vi "Poll PDOs.vi"(0 "interface object in":refnum<k20>, 1 "node-ID":u8=1, 11 "error in (no error)":errorcluster) -> (4 "PDO 1":u8[](array[numeric]), 6 "PDO 2":u8[](array[numeric]), 8 "PDO 3":u8[](array[numeric]), 10 "PDO 4":u8[](array[numeric]), 15 "error out":errorcluster)   [LabVIEW 2016]
uses:
  <vilib>/Platform/TimedLoop/XDataNode/timing_clust.ctl
  <vilib>/Platform/TimedLoop/XDataNode/nitl_modes.ctl
  <vilib>/Platform/TimedLoop/XDataNode/wakeup.ctl
  <vilib>/CANopenLib/CANOPEN.llb/CANopen SYNC Create.vi
  <vilib>/CANopenLib/CANOPEN.llb/CANopen SYNC Start.vi
  <vilib>/CANopenLib/CANOPEN.llb/CANopen TPDO Create.vi
  <vilib>/CANopenLib/CANOPEN.llb/CANopen TPDO Start.vi
  <vilib>/CANopenLib/CANOPEN.llb/CANopen SYNC Close.vi
  <vilib>/CANopenLib/CANOPEN.llb/CANopen TPDO Close.vi
  <vilib>/Platform/TimedLoop/XDataNode/XDataNode.xnode
  <vilib>/Platform/TimedLoop/XDataNode/XDNodeRunTimeDep.lvlib
panel:
  in  "counter overflow value":u8=5
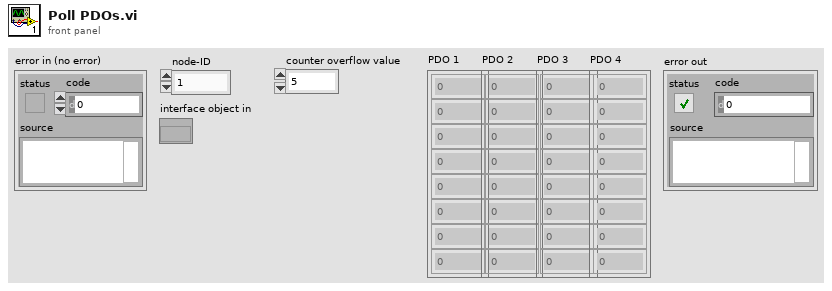
[diagram p1: front panel]
types:
  T1 = typedef "XDNodeRunTimeDep.lvlib/timing_clust.ctl" = cluster{"Expected End [f-1]":u64, "Actual End [f-1]":u64, "Finished Late? [f-1]":bool, "Expected End [i-1]":u64, "Actual End [i-1]":u64, "Finished Late? [i-1]":bool, "Expected Start [i]":u64, "Actual Start [i]":u64, "Expected Start [f]":u64, "Actual Start [f]":u64, "Source Name":string, "Structure Name":string, "Period":i64, "Deadline":i64, "Offset":i64, "Start":i64, "Priority":i32, "Timeout":i32, "Mode":T2, "Wakeup Reason":T3, "Error":errorcluster, "Source Type":string, "Secondary Source Type":string, "Global End Time":u64, "Global Start Time":u64, "Frame Duration":u64, "Iteration Duration":u64, "Assigned CPU":i32, "I/O Scan Engine Mode":u32}
  T2 = typedef "XDNodeRunTimeDep.lvlib/nitl_modes.ctl" = enum32{"No Change", "Process missed periods, maintain original phase", "Discard missed periods, maintain original phase", "Process missed periods, ignore original phase", "Discard missed periods, ignore original phase"}
  T3 = typedef "XDNodeRunTimeDep.lvlib/wakeup.ctl" = enum32{"Normal", "Aborted", "Asynchronous wakeup", "Timing source error", "Timed loop error", "Timeout"}
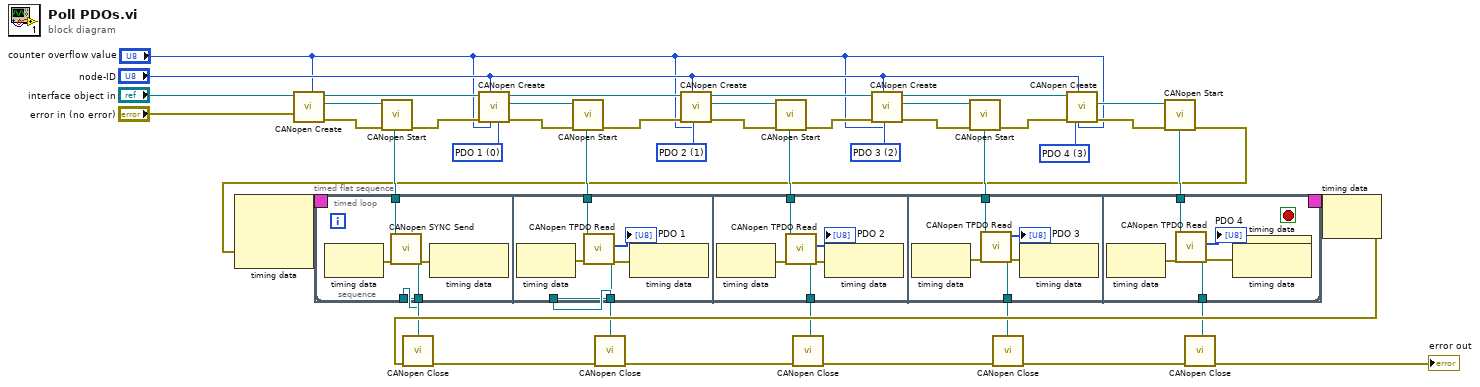
[diagram p0: block diagram]
diagram:
  w12 = u8 3 items=["PDO 1", "PDO 2", "PDO 3", "PDO 4"] ("PDO channel")
  w15 = u8 2 items=["PDO 1", "PDO 2", "PDO 3", "PDO 4"] ("PDO channel")
  w18 = u8 1 items=["PDO 1", "PDO 2", "PDO 3", "PDO 4"] ("PDO channel")
  w21 = u8 0 items=["PDO 1", "PDO 2", "PDO 3", "PDO 4"] ("PDO channel")
  n1 = call-poly <vilib>:"CANopen Create.vi"("error in (no error)"="error in (no error)", "counter overflow value (0)"="counter overflow value", "interface object in"="interface object in") -> ("error out"=w24:errorcluster, "SYNC object out"=w25:refnum<k20>, "interface object out"=w11:refnum<k20>)  [unwired: 6 in]
  n2 = call-poly <vilib>:"CANopen Start.vi"("error in (no error)"=w24, "SYNC object in"=w25) -> ("error out"=w7:errorcluster, "SYNC object out"=w42:refnum<k20>)  [unwired: 8 in]
  n3 = call-poly <vilib>:"CANopen Create.vi"("buffer size (0)"="counter overflow value", "node-ID"="node-ID", "error in (no error)"=w7, "PDO channel"=w21, "interface object in"=w11) -> ("error out"=w23:errorcluster, "TPDO object out"=w22:refnum<k20>, "interface object out"=w10:refnum<k20>)  [unwired: 4 in]
  n4 = call-poly <vilib>:"CANopen Start.vi"("error in (no error)"=w23, "TPDO object in"=w22) -> ("error out"=w6:errorcluster, "TPDO object out"=w40:refnum<k20>)  [unwired: 8 in]
  n5 = call-poly <vilib>:"CANopen Create.vi"("buffer size (0)"="counter overflow value", "node-ID"="node-ID", "error in (no error)"=w6, "PDO channel"=w18, "interface object in"=w10) -> ("error out"=w20:errorcluster, "TPDO object out"=w19:refnum<k20>, "interface object out"=w9:refnum<k20>)  [unwired: 4 in]
  n6 = call-poly <vilib>:"CANopen Start.vi"("error in (no error)"=w20, "TPDO object in"=w19) -> ("error out"=w5:errorcluster, "TPDO object out"=w37:refnum<k20>)  [unwired: 8 in]
  n7 = call-poly <vilib>:"CANopen Create.vi"("buffer size (0)"="counter overflow value", "node-ID"="node-ID", "error in (no error)"=w5, "PDO channel"=w15, "interface object in"=w9) -> ("error out"=w17:errorcluster, "TPDO object out"=w16:refnum<k20>, "interface object out"=w8:refnum<k20>)  [unwired: 4 in]
  n8 = call-poly <vilib>:"CANopen Start.vi"("error in (no error)"=w17, "TPDO object in"=w16) -> ("error out"=w4:errorcluster, "TPDO object out"=w36:refnum<k20>)  [unwired: 8 in]
  n9 = call-poly <vilib>:"CANopen Create.vi"("buffer size (0)"="counter overflow value", "node-ID"="node-ID", "error in (no error)"=w4, "PDO channel"=w12, "interface object in"=w8) -> ("error out"=w14:errorcluster, "TPDO object out"=w13:refnum<k20>)  [unwired: 4 in, 1 out]
  n10 = call-poly <vilib>:"CANopen Start.vi"("error in (no error)"=w14, "TPDO object in"=w13) -> ("error out"=w32:errorcluster, "TPDO object out"=w35:refnum<k20>)  [unwired: 8 in]
  n11 = node-c288(w32) -> (w45:T1)  [unwired: 2 in]
  n12 = timed-loop {
    timing: w45 -> [_]
    timing-out: [_] -> w44
    tunnel: w42 -> [w55]
    tunnel: w40 -> [w54]
    tunnel: [w53] -> w39
    tunnel: w37 -> [w52]
    tunnel: [w51] -> w38
    tunnel: w36 -> [w50]
    tunnel: w35 -> [w49]
    tunnel: [w48] -> w34
    tunnel: [w47] -> w33
    tunnel: [w46] -> w30
    stop <- _ stop-if-true
    n13 = timed-sequence {
      timing: _ -> [_]
      timing-out: _ -> [_]
      tunnel: w55 -> [w65]
      tunnel: w54 -> [w64]
      tunnel: [w63] -> w53
      tunnel: w52 -> [w62]
      tunnel: [w61] -> w51
      tunnel: w50 -> [w60]
      tunnel: w49 -> [w59]
      tunnel: [w58] -> w48
      tunnel: [w57] -> w47
      tunnel: [w56] -> w46
      n14 = timed-flat-sequence {
        tunnel: w65 -> [w69]
        tunnel: [w66] -> w56
        tunnel: w64 -> [w79]
        tunnel: [w78] -> w63
        tunnel: w62 -> [w86]
        tunnel: [w85] -> w61
        tunnel: w60 -> [w96]
        tunnel: [w95] -> w57
        tunnel: w59 -> [w107]
        tunnel: [w106] -> w58
        frame #0 {
          n15 = node-c288() -> (w68:errorcluster)  [unwired: 1 in]
          n16 = call <vilib>:"CANopen SYNC Send.vi"("error in (no error)"=w68, "SYNC object in"=w69) -> ("error out"=w67:errorcluster, "SYNC object out"=w66:refnum<k20>)  [unwired: 8 in]
          n17 = node-c288(w67) -> ()  [unwired: 1 out]
        }
        frame #1 {
          n18 = node-c288() -> (w77:errorcluster)  [unwired: 1 in]
          n19 = call <vilib>:"CANopen TPDO Read.vi"("error in (no error)"=w77, "TPDO object in"=w79) -> ("error out"=w76:errorcluster, "data"=→"PDO 1":u8[], "TPDO object out"=w78:refnum<k20>)  [unwired: 5 in, 2 out]
          n20 = node-c288(w76) -> ()  [unwired: 1 out]
        }
        frame #2 {
          n21 = node-c288() -> (w88:errorcluster)  [unwired: 1 in]
          n22 = call <vilib>:"CANopen TPDO Read.vi"("error in (no error)"=w88, "TPDO object in"=w86) -> ("error out"=w87:errorcluster, "data"=→"PDO 2":u8[], "TPDO object out"=w85:refnum<k20>)  [unwired: 5 in, 2 out]
          n23 = node-c288(w87) -> ()  [unwired: 1 out]
        }
        frame #3 {
          n24 = node-c288() -> (w98:errorcluster)  [unwired: 1 in]
          n25 = call <vilib>:"CANopen TPDO Read.vi"("error in (no error)"=w98, "TPDO object in"=w96) -> ("error out"=w97:errorcluster, "data"=→"PDO 3":u8[], "TPDO object out"=w95:refnum<k20>)  [unwired: 5 in, 2 out]
          n26 = node-c288(w97) -> ()  [unwired: 1 out]
        }
        frame #4 {
          n27 = node-c288() -> (w108:errorcluster)  [unwired: 1 in]
          n28 = call <vilib>:"CANopen TPDO Read.vi"("error in (no error)"=w108, "TPDO object in"=w107) -> ("error out"=w105:errorcluster, "data"=→"PDO 4":u8[], "TPDO object out"=w106:refnum<k20>)  [unwired: 5 in, 2 out]
          n29 = node-c288(w105) -> ()  [unwired: 1 out]
        }
      }
    }
    n30 = node-c288() -> ()  [unwired: 1 in, 1 out]
    n31 = node-c288() -> ()  [unwired: 1 in, 1 out]
  }
  n32 = node-c288(w44) -> (w41:errorcluster)
  n33 = call-poly <vilib>:"CANopen Close.vi"("error in (no error)"=w41, "SYNC object in"=w30) -> ("error out"=w31:errorcluster)  [unwired: 9 in]
  n34 = call-poly <vilib>:"CANopen Close.vi"("error in (no error)"=w31, "TPDO object in"=w39) -> ("error out"=w29:errorcluster)  [unwired: 9 in]
  n35 = call-poly <vilib>:"CANopen Close.vi"("error in (no error)"=w29, "TPDO object in"=w38) -> ("error out"=w28:errorcluster)  [unwired: 9 in]
  n36 = call-poly <vilib>:"CANopen Close.vi"("error in (no error)"=w28, "TPDO object in"=w33) -> ("error out"=w27:errorcluster)  [unwired: 9 in]
  n37 = call-poly <vilib>:"CANopen Close.vi"("error in (no error)"=w27, "TPDO object in"=w34) -> ("error out"=→"error out":errorcluster)  [unwired: 9 in]
